vi "CelsiusToOthers.vi"() -> ()   [LabVIEW 2020]
panel:
  out "Fahrenheit":dbl
  out "Kelvin":dbl
  in  "Celsius":dbl
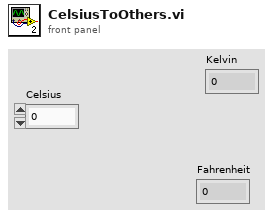
[diagram p1: front panel]
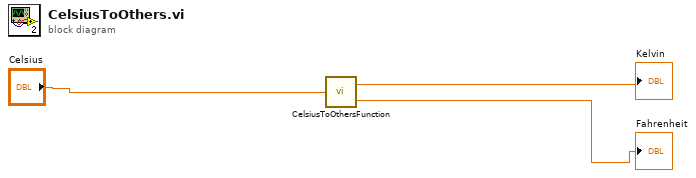
[diagram p0: block diagram]
diagram:
  n1 = call "CelsiusToOthersFunction.vi"("Celsius"="Celsius") -> ("k"=→"Kelvin":dbl, "f"=→"Fahrenheit":dbl)
